vi "users save user.vi"(6 "Current User":T1, 8 "error in (no error)":errorcluster, 9 "Username (\"\")":string, 10 "POST (empty)":T2, 11 "Connection Ref":T3) -> (0 "error out":errorcluster, 1 "User Credentials Change?":bool, 2 "new User Record":T1, 3 "dup Connection Ref":T3, 4 "Current Record Edit?":bool)   [LabVIEW 2011]
uses:
  SI.LIB/ODBC/SQL Controls/Connection Refnum.ctl
  server/database/Users/User Record.ctl
  Addons/internet/utils/keyedarr.llb/Keyed Array.ctl
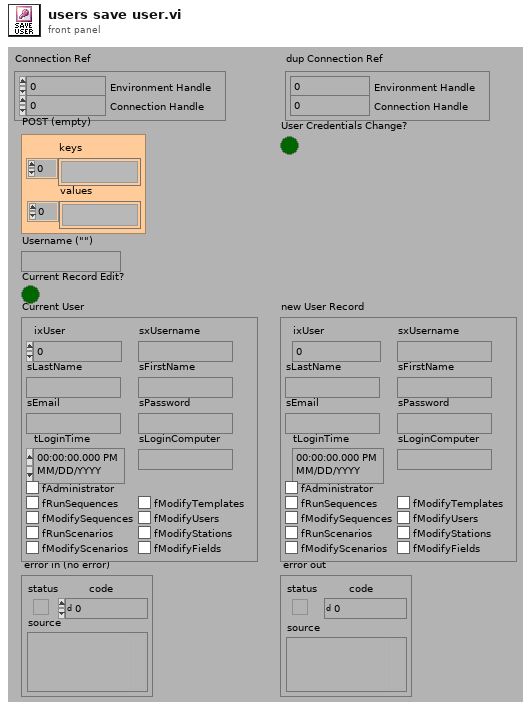
[diagram p1: front panel]
types:
  T1 = typedef "User Record.ctl" = cluster{"ixUser":i32, "sxUsername":string, "sLastName":string, "sFirstName":string, "sEmail":string, "sPassword":string, "tLoginTime":timestamp, "sLoginComputer":string, "fAdministrator":bool, "fRunSequences":bool, "fModifySequences":bool, "fRunScenarios":bool, "fModifyScenarios":bool, "fModifyTemplates":bool, "fModifyUsers":bool, "fModifyStations":bool, "fModifyFields":bool}
  T2 = typedef "Keyed Array.ctl" = cluster{"keys":string[], "values":string[]}
  T3 = typedef "Connection Refnum.ctl" = cluster{"Environment Handle":i32, "Connection Handle":i32}
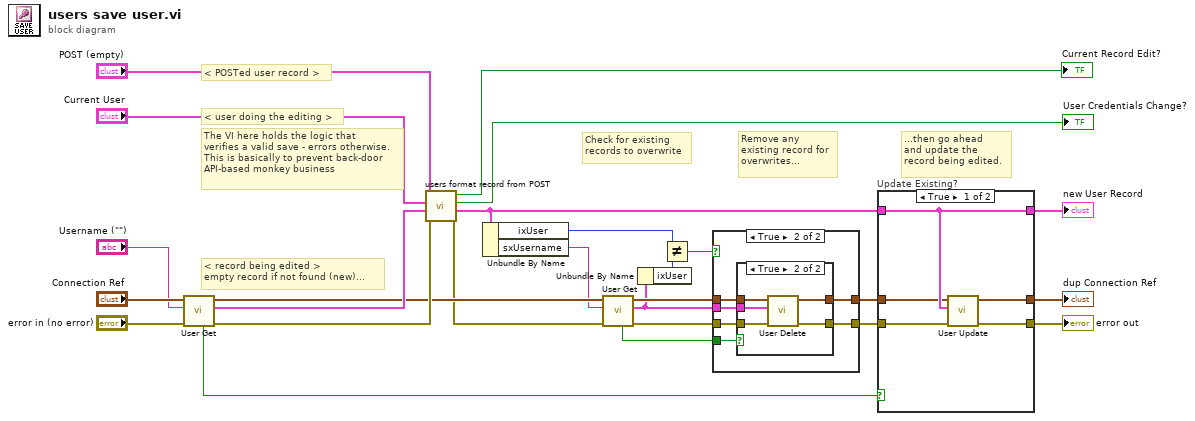
[diagram p0: block diagram]
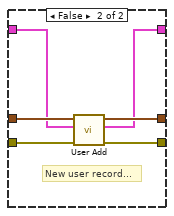
[diagram p4: hidden frame]
diagram:
  # "...then go ahead\nand update the\nrecord being edited."
  # "Check for existing\nrecords to overwrite"
  # "Remove any\nexisting record for\noverwrites..."
  # "The VI here holds the logic that\nverifies a valid save - errors otherwise.\nThis is basically to prevent back-door\nAPI-based monkey business"
  # "< POSTed user record >"
  # "< user doing the editing >"
  # "< record being edited >\nempty record if not found (new)..."
  n1 = call "User Get.vi"("error in (no error)"="error in (no error)", "sxUsername (\"\")"="Username (\"\")", "Connection Refnum"="Connection Ref") -> ("error out"=w18:errorcluster, "User"=w14:T1, "Connection Refnum"=w13:T3, "Data Present?"=w15:bool)  [unwired: 5 out]
  n2 = call "users format record from POST.vi"("error in (no error)"=w18, "Edited User (none)"=w14, "Current User (none)"="Current User", "POST (empty)"="POST (empty)") -> ("error out"=w10:errorcluster, "Record to Commit"=w12:T1, "Current User Credential Change?"=→"User Credentials Change?":bool, "Current Record Edit?"=→"Current Record Edit?":bool)  [unwired: 4 out]
  n3 = Unbundle By Name(w12) -> ("ixUser"=w8:i32, "sxUsername"=w11:string)
  n4 = call "User Get.vi"("error in (no error)"=w10, "sxUsername (\"\")"=w11, "Connection Refnum"=w13) -> ("error out"=w6:errorcluster, "User"=w1:T1, "Connection Refnum"=w7:T3, "Data Present?"=w3:bool)  [unwired: 5 out]
  n5 = Unbundle By Name(w1) -> ("ixUser"=w9:i32)
  n6 = Not Equal?(x=w8, y=w9) -> (x != y?=w2:bool)
  n7 = case shown="True" w2 {
    tunnel: [w28 w34] -> w5
    tunnel: [w27 w33] -> w4
    tunnel: w1 -> [_ w32]
    tunnel: w6 -> [w27 w31]
    tunnel: w7 -> [w28 w30]
    tunnel: w3 -> [_ w29]
    frame False {
    }
    frame True {
      n8 = case shown="True" w29 {
        tunnel: w30 -> [w36 w41]
        tunnel: [w36 w40] -> w34
        tunnel: w31 -> [w35 w39]
        tunnel: w32 -> [_ w38]
        tunnel: [w35 w37] -> w33
        frame False {
        }
        frame True {
          n9 = call "User Delete.vi"("error in (no error)"=w39, "User Record"=w38, "Connection Refnum"=w41) -> ("error out"=w37:errorcluster, "Connection Refnum"=w40:T3)  [unwired: 7 out]
        }
      }
    }
  }
  n10 = case "Update Existing?" shown="True" w15 {
    tunnel: w4 -> [w42 w52]
    tunnel: [w45 w51] -> w22
    tunnel: [w46 w49] -> w26
    tunnel: w5 -> [w43 w50]
    tunnel: [w44 w48] -> w25
    tunnel: w12 -> [w44 w47]
    frame True {
      n11 = call "User Update.vi"("error in (no error)"=w42, "User Record"=w44, "Connection Refnum"=w43) -> ("error out"=w45:errorcluster, "dup Connection Refnum"=w46:T3)  [unwired: 7 out]
    }
    frame False {
      # "New user record..."
      n12 = call "User Add.vi"("error in (no error)"=w52, "User Record"=w47, "Connection Refnum"=w50) -> ("error out"=w51:errorcluster, "New User Record"=w48:T1, "Connection Refnum"=w49:T3)  [unwired: 6 out]
    }
  }
  "error out" <- w22
  "dup Connection Ref" <- w26
  "new User Record" <- w25
